vi "SD-Color Table Generator.vi"() -> (0 "?":u32[](array[colorbox])=[0, 16711680, 16646657, 16516097, 16451074, 16386051, 16255491, 16190468, 16059909, 15994885, 15929862, 15799303, 15734279, 15669256, 15538697, 15473674, 15408650, 15278091, 15213068, 15082508, 15017485, 14952462, 14821902, 14756879, 14691856, 14561296, 14496273, 14431250, 14300690, 14235667, 14105108, 14040084, 13975061, 13844502, 13779478, 13714455, 13583896, 13518872, 13453849, 13323290, 13258267, 13127707, 13062684, 12997661, 12867101, 12802078, 12737055, 12606495, 12541472, 12476449, 12345889, 12280866, 12150307, 12085283, 12020260, 11889701, 11824677, 11759654, 11629095, 11564071, 11499048, 11368489, 11303465, 11172906, 11107883, 11043116, 10912556, 10847533, 10782510, 10651950, 10586927, 10456368, 10391344, 10326321, 10195762, 10130738, 10065715, 9935156, 9870132, 9805109, 9674550, 9609526, 9478967, 9413944, 9348920, 9218361, 9153338, 9088314, 8957755, 8892732, 8827709, 8697149, 8632126, 8501567, 8436543, 8371520, 8240961, 8175937, 8110914, 7980355, 7915331, 7850308, 7719749, 7654725, 7524166, 7459143, 7394119, 7263560, 7198537, 7133513, 7002954, 6937931, 6872907, 6742348, 6677325, 6546766, 6481742, 6416719, 6286160, 6221136, 6156113, 6025554, 5960530, 5895507, 5764948, 5699924, 5569365, 5504342, 5439320, 5307737, 5241690, 5175644, 5175133, 5109086, 5043040, 5042529, 4976482, 4975972, 4909925, 4843878, 4843368, 4777321, 4711274, 4710764, 4644717, 4578670, 4578160, 4512113, 4511602, 4445300, 4379253, 4378742, 4312696, 4246649, 4246138, 4180092, 4114045, 4113534, 4047488, 4046977, 3980930, 3914883, 3914373, 3848326, 3782279, 3781769, 3715722, 3649675, 3649165, 3583118, 3582607, 3516561, 3450514, 3450003, 3383957, 3317910, 3317399, 3251353, 3185306, 3184795, 3118749, 3118238, 3052191, 2986145, 2985634, 2919587, 2853541, 2853030, 2786983, 2720937, 2720426, 2654379, 2588077, 2587566, 2521519, 2521009, 2454962, 2388915, 2388405, 2322358, 2256311, 2255801, 2189754, 2123707, 2123197, 2057150, 2056639, 1990593, 1924546, 1924035, 1857989, 1791942, 1791431, 1725385, 1659338, 1658827, 1592781, 1592270, 1526223, 1460177, 1459666, 1393619, 1327573, 1327062, 1261015, 1194968, 1194458, 1128411, 1127900, 1061854, 995807, 995296, 929250, 863203, 862436, 796390, 730343, 729832, 663786, 663275, 597228, 531182, 530671, 464624, 398578, 398067, 332020, 265974, 265463, 199416, 198906, 132859, 66812, 66302, 255, 16711680], 1 "Cancel 2":bool)   [LabVIEW 2020]
doc: "Color Table Generator.vi is a subVI called by Color Table Example.vi\n\nThis VI generates a color table based on the beginning, middle, and end RGB color combinations the user specifies. Using an XY graph and cursors, the user mixes red, green, and blue components to create the start, middle, and end color combinations for the color table."
panel:
  in  "Out of range below\n(color 0)":u32(colorbox)
  in  "Out of range above\n(color 255)":u32(colorbox)=16711680
  in  "Cancel":bool
  in  "Accept":bool
  in  "final color":cluster{u8, u8, u8}(slide)={0, 0, 255} scale=0.0..255.0
  in  "beginning color":cluster{u8, u8, u8}(slide)={255, 0, 0} scale=0.0..255.0
  out "?":cluster{u8[]}[](graph)=[{[255, 254, 252, 251, 250, 248, 247, 245, 244, 243, 241, 240, 239, 237, 236, 235, 233, 232, 230, 229, 228, 226, 225, 224, 222, 221, 220, 218, 217, 215, 214, 213, 211, 210, 209, 207, 206, 205, 203, 202, 200, 199, 198, 196, 195, 194, 192, 191, 190, 188, 187, 185, 184, 183, 181, 180, 179, 177, 176, 175, 173, 172, 170, 169, 168, 166, 165, 164, 162, 161, 159, 158, 157, 155, 154, 153, 151, 150, 149, 147, 146, 144, 143, 142, 140, 139, 138, 136, 135, 134, 132, 131, 129, 128, 127, 125, 124, 123, 121, 120, 119, 117, 116, 114, 113, 112, 110, 109, 108, 106, 105, 104, 102, 101, 99, 98, 97, 95, 94, 93, 91, 90, 89, 87, 86, 84, 83, 82, 80, 79, 78, 78, 77, 76, 76, 75, 75, 74, 73, 73, 72, 71, 71, 70, 69, 69, 68, 68, 67, 66, 66, 65, 64, 64, 63, 62, 62, 61, 61, 60, 59, 59, 58, 57, 57, 56, 55, 55, 54, 54, 53, 52, 52, 51, 50, 50, 49, 48, 48, 47, 47, 46, 45, 45, 44, 43, 43, 42, 41, 41, 40, 39, 39, 38, 38, 37, 36, 36, 35, 34, 34, 33, 32, 32, 31, 31, 30, 29, 29, 28, 27, 27, 26, 25, 25, 24, 24, 23, 22, 22, 21, 20, 20, 19, 18, 18, 17, 17, 16, 15, 15, 14, 13, 13, 12, 11, 11, 10, 10, 9, 8, 8, 7, 6, 6, 5, 4, 4, 3, 3, 2, 1, 1, 0]}, {[0, 2, 4, 6, 8, 10, 12, 14, 16, 18, 20, 22, 24, 26, 28, 30, 32, 34, 36, 38, 40, 42, 44, 46, 48, 50, 52, 54, 56, 58, 60, 62, 64, 66, 68, 70, 72, 74, 76, 78, 80, 82, 84, 86, 88, 90, 92, 94, 96, 98, 100, 102, 104, 106, 108, 110, 112, 114, 116, 118, 120, 122, 124, 126, 129, 131, 133, 135, 137, 139, 141, 143, 145, 147, 149, 151, 153, 155, 157, 159, 161, 163, 165, 167, 169, 171, 173, 175, 177, 179, 181, 183, 185, 187, 189, 191, 193, 195, 197, 199, 201, 203, 205, 207, 209, 211, 213, 215, 217, 219, 221, 223, 225, 227, 229, 231, 233, 235, 237, 239, 241, 243, 245, 247, 249, 251, 253, 255, 253, 251, 249, 247, 245, 243, 241, 239, 237, 235, 233, 231, 229, 227, 225, 223, 221, 219, 217, 215, 212, 210, 208, 206, 204, 202, 200, 198, 196, 194, 192, 190, 188, 186, 184, 182, 180, 178, 176, 174, 172, 170, 168, 166, 164, 162, 160, 158, 156, 154, 152, 150, 148, 146, 144, 142, 140, 138, 136, 134, 132, 130, 128, 125, 123, 121, 119, 117, 115, 113, 111, 109, 107, 105, 103, 101, 99, 97, 95, 93, 91, 89, 87, 85, 83, 81, 79, 77, 75, 73, 71, 69, 67, 65, 63, 61, 59, 57, 55, 53, 51, 49, 47, 45, 43, 40, 38, 36, 34, 32, 30, 28, 26, 24, 22, 20, 18, 16, 14, 12, 10, 8, 6, 4, 2, 0]}, {[0, 1, 1, 2, 3, 3, 4, 5, 5, 6, 7, 7, 8, 9, 10, 10, 11, 12, 12, 13, 14, 14, 15, 16, 16, 17, 18, 18, 19, 20, 20, 21, 22, 22, 23, 24, 24, 25, 26, 27, 27, 28, 29, 29, 30, 31, 31, 32, 33, 33, 34, 35, 35, 36, 37, 37, 38, 39, 39, 40, 41, 41, 42, 43, 44, 44, 45, 46, 46, 47, 48, 48, 49, 50, 50, 51, 52, 52, 53, 54, 54, 55, 56, 56, 57, 58, 58, 59, 60, 61, 61, 62, 63, 63, 64, 65, 65, 66, 67, 67, 68, 69, 69, 70, 71, 71, 72, 73, 73, 74, 75, 75, 76, 77, 78, 78, 79, 80, 80, 81, 82, 82, 83, 84, 84, 85, 86, 88, 89, 90, 92, 93, 94, 96, 97, 98, 100, 101, 102, 104, 105, 106, 108, 109, 110, 112, 113, 114, 116, 117, 118, 120, 121, 122, 124, 125, 126, 128, 129, 130, 131, 133, 134, 135, 137, 138, 139, 141, 142, 143, 145, 146, 147, 149, 150, 151, 153, 154, 155, 157, 158, 159, 161, 162, 163, 165, 166, 167, 169, 170, 171, 173, 174, 175, 177, 178, 179, 181, 182, 183, 185, 186, 187, 189, 190, 191, 193, 194, 195, 197, 198, 199, 201, 202, 203, 205, 206, 207, 209, 210, 211, 213, 214, 215, 216, 218, 219, 220, 222, 223, 224, 226, 227, 228, 230, 231, 232, 234, 235, 236, 238, 239, 240, 242, 243, 244, 246, 247, 248, 250, 251, 252, 254, 255]}]
  # "Use the two sliders\nand the cursors to\ndefine the color table."
  # "Color wieghts for RGB"
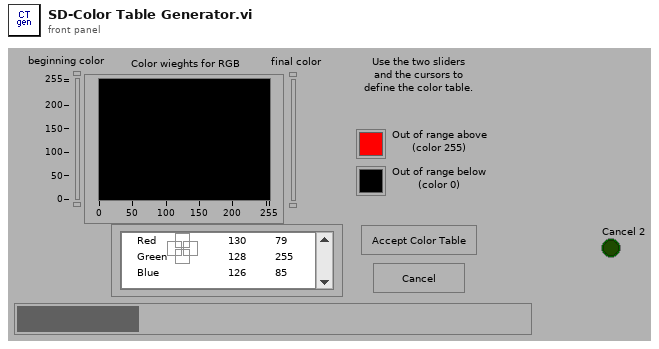
[diagram p1: front panel]
types:
  T1 = cluster{u8, u8, "Cursor.Cursor Y":dbl, "Cursor.Cursor X":dbl}
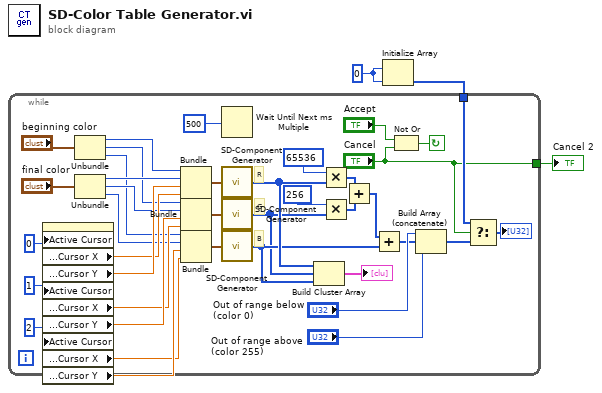
[diagram p0: block diagram]
diagram:
  w3 = u32 0
  n1 = Initialize Array(w3, w3) -> (w2:u32[])
  n2 = while {
    tunnel: w2 -> [w15]
    tunnel: ["Cancel"] -> w1
    stop <- w16 continue-if-true
    # "B"
    # "G"
    # "R"
    n3 = property class="WFGraph (strict)"("Active Cursor"=0, "Active Cursor"=1, "Active Cursor"=2) -> ("Cursor.Cursor Position:Cursor X"=w37:dbl, "Cursor.Cursor Position:Cursor Y"=w38:dbl, "Cursor.Cursor Position:Cursor X"=w39:dbl, "Cursor.Cursor Position:Cursor Y"=w40:dbl, "Cursor.Cursor Position:Cursor X"=w41:dbl, "Cursor.Cursor Position:Cursor Y"=w42:dbl)  [unwired: 2 in, 2 out]
    n4 = Unbundle("beginning color") -> (w31:u8, w32:u8, w33:u8)
    n5 = Unbundle("final color") -> (w34:u8, w35:u8, w36:u8)
    n6 = Bundle(w31, w34, "Cursor.Cursor Y"=w38, "Cursor.Cursor X"=w37) -> (w28:T1)  [unwired: 1 in]
    n7 = Bundle(w32, w35, "Cursor.Cursor Y"=w40, "Cursor.Cursor X"=w39) -> (w12:T1)  [unwired: 1 in]
    n8 = Bundle(w33, w36, "Cursor.Cursor Y"=w42, "Cursor.Cursor X"=w41) -> (w11:T1)  [unwired: 1 in]
    n9 = Wait Until Next ms Multiple(millisecond multiple=500) -> ()  [unwired: 1 out]
    n10 = call "SD-Component Generator.vi"("Component definition"=w28) -> ("Component array"=w24:u8[])
    n11 = call "SD-Component Generator.vi"("Component definition"=w12) -> ("Component array"=w9:u8[])
    n12 = call "SD-Component Generator.vi"("Component definition"=w11) -> ("Component array"=w10:u8[])
    n13 = Build Cluster Array(w24, w9, w10) -> (→"?":cluster{"Component array":u8[]}[])
    n14 = Multiply(x=u32 65536, y=w24) -> (x*y=w21:u32[])
    n15 = Multiply(x=u32 256, y=w9) -> (x*y=w20:u32[])
    n16 = Add(x=w21, y=w20) -> (x+y=w22:u32[])
    n17 = Add(x=w22, y=w10) -> (x+y=w5:u32[])
    n18 = Not Or(1:"Cancel", 2:"Accept") -> (0:w16:bool)
    n19 = Build Array (concatenate)("Out of range below\n(color 0)", w5, "Out of range above\n(color 255)") -> (w8:u32[])
    n20 = Select(t=w15, s="Cancel", f=w8) -> (s? t:f=→"?":u32[])
  }
  "Cancel 2" <- w1
